vi "Set Master-Slave Jog Velocity Update Interval.vi"(4 "error in (no error)":errorcluster, 6 "Interval":i32=1 min=1 max=1000, 7 "VISA resource name":refnum<visa-resource-name>) -> (0 "error out":errorcluster, 3 "VISA resource name out":refnum<visa-resource-name>)   [LabVIEW 2014, in "Newport ESP301.lvlib"]
doc: "This command sets the jog velocity update interval for slave axis. The jog velocity of slave axis is computed once every interval using user specified scaling coefficients and the master axis velocity at the time of computation. Refer SK command to specify slave jog velocity scaling coefficients. Note that appropriate trajectory mode has to be specified using TJ command before this command becomes effective."
uses:
  Newport ESP301.lvlib
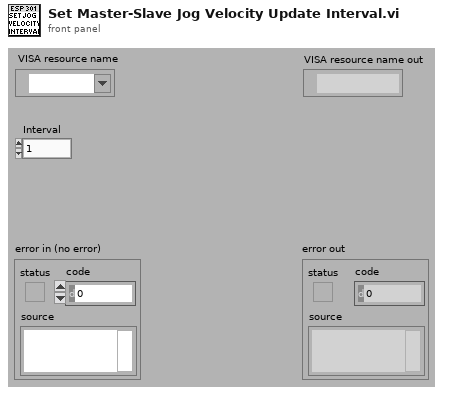
[diagram p1: front panel]
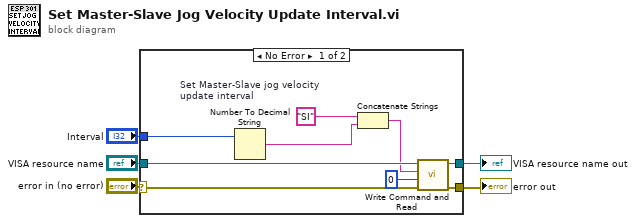
[diagram p0: block diagram]
diagram:
  n1 = case shown="No Error" "error in (no error)" {
    selector: "error in (no error)" -> [w10 w16]
    tunnel: [w8 w16] -> w5
    tunnel: "VISA resource name" -> [w13 w15]
    tunnel: [w9 w15] -> w4
    tunnel: "Interval" -> [w6 _]
    frame No Error {
      w14 = "SI"  # Set Master-Slave jog velocity update interval
      n2 = Number To Decimal String(number=w6) -> (decimal integer string=w7:string)  [unwired: 1 out]
      n3 = Concatenate Strings(w14, w7) -> (w12:string)
      n4 = call "Write Command and Read.vi"("error in (no error)"=w10, "Bytes to read (100)"=u32 0, "Command"=w12, "VISA resource name"=w13) -> ("error out"=w8:errorcluster, "VISA resource name out"=w9:refnum<visa-resource-name>)  [unwired: 1 in, 3 out]
    }
    frame Error {
    }
  }
  "error out" <- w5
  "VISA resource name out" <- w4
